vi "FFT_comparison_vi_vs_impl.vi"() -> ()   [LabVIEW 2025]
uses:
  <vilib>/Analysis/2dsp.llb/Real FFT.vi
  <vilib>/Analysis/NI_AALPro.lvlib
panel:
  out "FFT{x}":cdb[](array[numeric])
  out "FFT {X}":cdb[](array[numeric])
  in  "Array":dbl[](array[numeric])
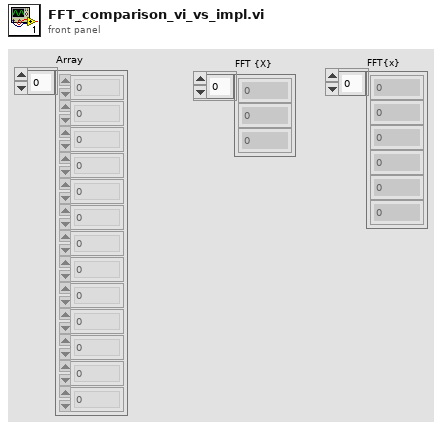
[diagram p1: front panel]
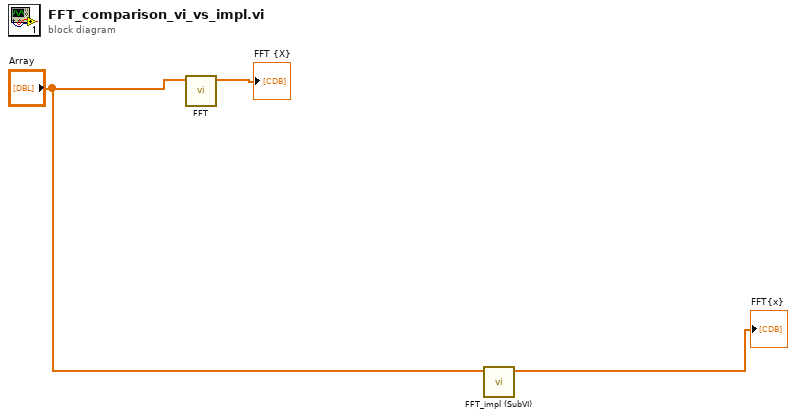
[diagram p0: block diagram]
diagram:
  n1 = call-poly <vilib>:"FFT.vi"("X"="Array") -> ("FFT {X}"=→"FFT {X}":cdb[])  [unwired: 9 in, 1 out]
  n2 = call "FFT_impl (SubVI).vi"("Array"="Array") -> ("FFT{x}"=→"FFT{x}":cdb[])  [unwired: 10 in]
